vi "Angle_Pid_Control.vi"(8 "desired module states":T1[](array[typedef]) {"Angle"."SIN" format="%13.4f"; "Angle"."COS" format="%13.4f"; "Angle"."VALUE" format="%13.4f"}, 9 "Current States":T1[](array[typedef]) {"Angle"."SIN" format="%13.4f"; "Angle"."COS" format="%13.4f"; "Angle"."VALUE" format="%13.4f"}) -> (2 "Vel Motor values":dbl[](array[numeric]), 3 "Angle Motor values":dbl[](array[numeric]))   [LabVIEW 2020]
doc: "takes the current and desired states and module id for the module and find the shortest distance traveled then calculates the motor control value for that angle motor"
uses:
  <vilib>/Rock Robotics/WPI/ThirdParty/JAS_Junk/TrajLib/TypeDef/SWERVE_DRIVE_MODULE_STATE.ctl
  <vilib>/Rock Robotics/WPI/ThirdParty/JAS_Junk/TrajLib/TypeDef/ROTATION2D.ctl
  <vilib>/Rock Robotics/WPI/ThirdParty/JAS_Junk/TrajLib/Rotation2d_Minus.vi
  <vilib>/Rock Robotics/WPI/ThirdParty/JAS_Junk/TrajLib/Rotation2d_GetRadians.vi
  <vilib>/Rock Robotics/WPI/ThirdParty/JAS_Junk/TrajLib/SwerveModuleState_New.vi
  <vilib>/Rock Robotics/WPI/ThirdParty/JAS_Junk/TrajLib/Rotation2d_RotateBy.vi
  <vilib>/Rock Robotics/WPI/ThirdParty/JAS_Junk/TrajLib/Rotation2d_CreateAngle.vi
  <vilib>/Rock Robotics/WPI/ThirdParty/JAS_Junk/TrajLib/Rotation2d_UnaryMinus.vi
  <vilib>/Rock Robotics/WPI/ThirdParty/JAS_Junk/TrajLib/Rotation2d_CreateXY.vi
  <vilib>/Rock Robotics/WPI/ThirdParty/JAS_Junk/TrajLib/Util_CalcDist.vi
  <vilib>/Rock Robotics/WPI/ThirdParty/JAS_Junk/TrajLib/Trajectory_Library.lvlib
panel:
  out "Angle Control Variable3 2":dbl
  out "Angle Control Variable3":dbl
  out "Angle Control Variable 2":dbl
  out "Angle Control Variable":dbl
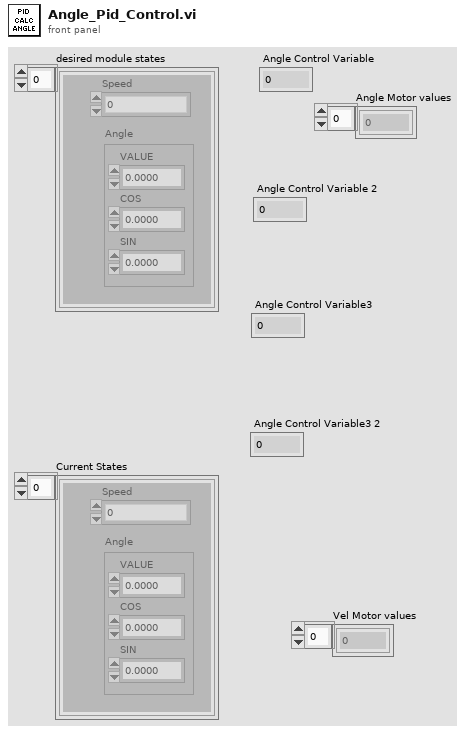
[diagram p1: front panel]
types:
  T1 = typedef "Trajectory_Library.lvlib/SWERVE_DRIVE_MODULE_STATE.ctl" = cluster{"Speed":dbl, "Angle":T2}
  T2 = typedef "Trajectory_Library.lvlib/ROTATION2D.ctl" = cluster{"VALUE":dbl, "COS":dbl, "SIN":dbl}
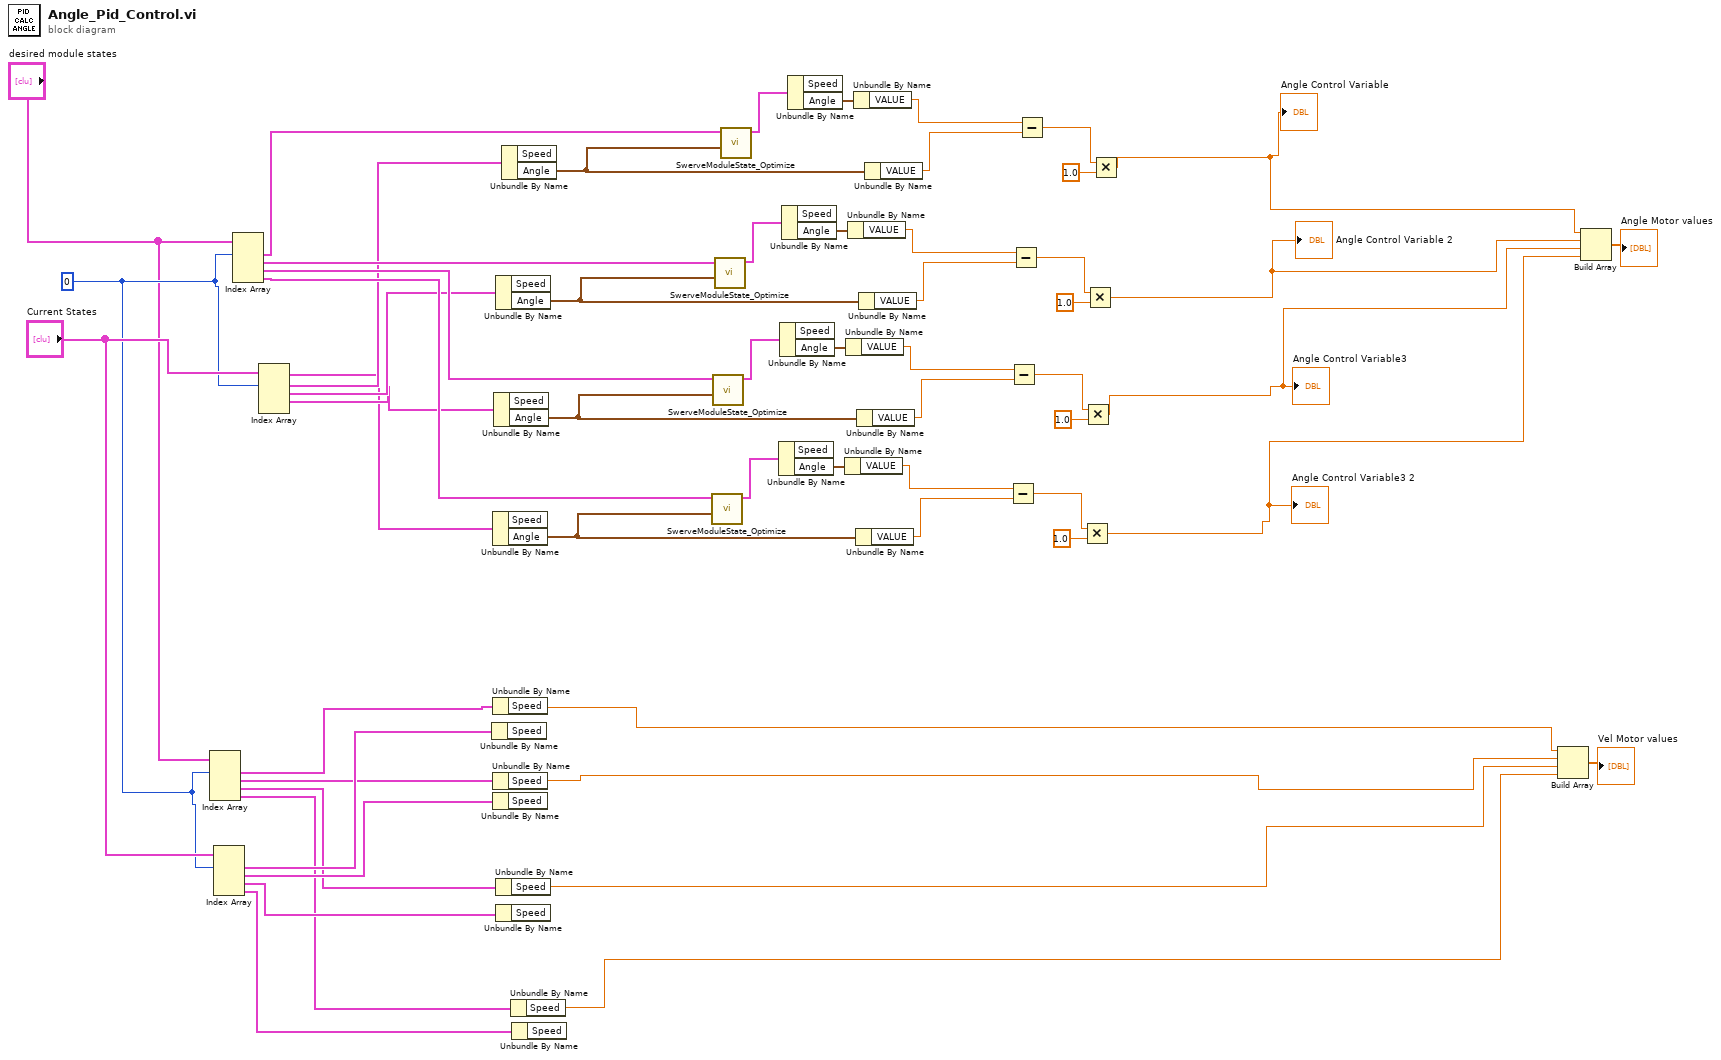
[diagram p0: block diagram]
diagram:
  w17 = 0 ("index")
  n1 = Index Array(array="desired module states", index #1=w17) -> (element #1=w15:T1, element #2=w14:T1, element #3=w12:T1, element #4=w9:T1)  [unwired: 3 in]
  n2 = Index Array(array="Current States", index #1=w17) -> (element #1=w19:T1, element #2=w13:T1, element #3=w11:T1, element #4=w10:T1)  [unwired: 3 in]
  n3 = Index Array(array="desired module states", index #1=w17) -> (element #1=w50:T1, element #2=w28:T1, element #3=w27:T1, element #4=w26:T1)  [unwired: 3 in]
  n4 = Index Array(array="Current States", index #1=w17) -> (element #1=w24:T1, element #2=w25:T1, element #3=w23:T1, element #4=w22:T1)  [unwired: 3 in]
  n5 = Unbundle By Name(w19) -> ()  [unwired: 1 out]
  n6 = Unbundle By Name(w22) -> ("Angle"=w33:T2)  [unwired: 1 out]
  n7 = Unbundle By Name(w15) -> ("Speed"=w4:dbl)
  n8 = Unbundle By Name(w14) -> ("Speed"=w3:dbl)
  n9 = Unbundle By Name(w13) -> ()  [unwired: 1 out]
  n10 = Unbundle By Name(w23) -> ("Angle"=w38:T2)  [unwired: 1 out]
  n11 = Unbundle By Name(w25) -> ("Angle"=w47:T2)  [unwired: 1 out]
  n12 = Unbundle By Name(w12) -> ("Speed"=w2:dbl)
  n13 = Unbundle By Name(w11) -> ()  [unwired: 1 out]
  n14 = Unbundle By Name(w24) -> ("Angle"=w53:T2)  [unwired: 1 out]
  n15 = Unbundle By Name(w9) -> ("Speed"=w1:dbl)
  n16 = Unbundle By Name(w10) -> ()  [unwired: 1 out]
  n17 = call <vilib>:"SwerveModuleState_Optimize.vi"("CurrentAngle"=w33, "Desired State"=w26) -> ("out SWERVE_DRIVE_MODULE_STATE"=w34:T1)  [unwired: 9 in]
  n18 = call <vilib>:"SwerveModuleState_Optimize.vi"("CurrentAngle"=w38, "Desired State"=w27) -> ("out SWERVE_DRIVE_MODULE_STATE"=w37:T1)  [unwired: 9 in]
  n19 = call <vilib>:"SwerveModuleState_Optimize.vi"("CurrentAngle"=w47, "Desired State"=w28) -> ("out SWERVE_DRIVE_MODULE_STATE"=w48:T1)  [unwired: 9 in]
  n20 = call <vilib>:"SwerveModuleState_Optimize.vi"("CurrentAngle"=w53, "Desired State"=w50) -> ("out SWERVE_DRIVE_MODULE_STATE"=w52:T1)  [unwired: 9 in]
  n21 = Unbundle By Name(w34) -> ("Angle"=w35:T2)  [unwired: 1 out]
  n22 = Unbundle By Name(w37) -> ("Angle"=w36:T2)  [unwired: 1 out]
  n23 = Unbundle By Name(w48) -> ("Angle"=w49:T2)  [unwired: 1 out]
  n24 = Unbundle By Name(w52) -> ("Angle"=w51:T2)  [unwired: 1 out]
  n25 = Unbundle By Name(w35) -> ("VALUE"=w32:dbl)
  n26 = Unbundle By Name(w36) -> ("VALUE"=w39:dbl)
  n27 = Unbundle By Name(w49) -> ("VALUE"=w46:dbl)
  n28 = Unbundle By Name(w51) -> ("VALUE"=w54:dbl)
  n29 = Unbundle By Name(w33) -> ("VALUE"=w31:dbl)
  n30 = Unbundle By Name(w38) -> ("VALUE"=w40:dbl)
  n31 = Unbundle By Name(w47) -> ("VALUE"=w45:dbl)
  n32 = Unbundle By Name(w53) -> ("VALUE"=w55:dbl)
  n33 = Subtract(x=w32, y=w31) -> (x-y=w30:dbl)
  n34 = Subtract(x=w39, y=w40) -> (x-y=w41:dbl)
  n35 = Subtract(x=w46, y=w45) -> (x-y=w44:dbl)
  n36 = Subtract(x=w54, y=w55) -> (x-y=w56:dbl)
  n37 = Multiply(x=w30, y=1.0) -> (x*y=w5:dbl)
  "Angle Control Variable3 2" <- w5
  n38 = Multiply(x=w41, y=1.0) -> (x*y=w6:dbl)
  "Angle Control Variable3" <- w6
  n39 = Multiply(x=w44, y=1.0) -> (x*y=w7:dbl)
  "Angle Control Variable 2" <- w7
  n40 = Multiply(x=w56, y=1.0) -> (x*y=w8:dbl)
  "Angle Control Variable" <- w8
  n41 = Build Array(w4, w3, w2, w1) -> (→"Vel Motor values":dbl[])
  n42 = Build Array(w8, w7, w6, w5) -> (→"Angle Motor values":dbl[])
